vi "grabAcquire_action.vi"(0 "HGF_ImaqDx":refnum<class "HGF_ImaqDx.lvclass">, 2 "Image In":T1, 3 "Wait for Next Buffer? (Yes)":bool=TRUE, 5 "error in (no error)":errorcluster) -> (14 "dup HGF_ImaqDx":refnum<class "HGF_ImaqDx.lvclass">, 16 "Image Out":T1, 17 "Acquired Buffer Number":u32, 19 "error out":errorcluster)   [LabVIEW 2014, in "HGF_IMAQ.lvlib" / "HGF_ImaqDx.lvclass"]
doc: "Acquires an image from a grab acquisition. Use the grab function for high-speed image acquisition.\n\nWait parameter is ignored by IMAQ for USB."
uses:
  HGF_ImaqDx.lvclass
  <vilib>/vision/Image Controls.llb/IMAQ Image.ctl
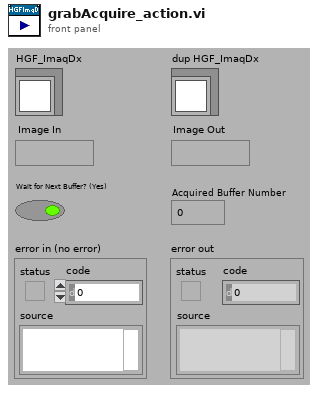
[diagram p1: front panel]
types:
  T1 = typedef "IMAQ Image.ctl" = refnum<image>
  T2 = typedef "IMAQdx.ctl" = refnum<k21>
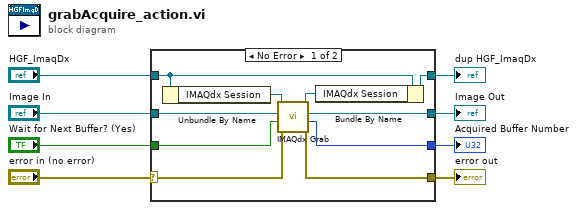
[diagram p0: block diagram]
diagram:
  n1 = case shown="No Error" "error in (no error)" {
    selector: "error in (no error)" -> [w9 w19]
    tunnel: "Image In" -> [w18 w20]
    tunnel: [w17 w20] -> w7
    tunnel: "Wait for Next Buffer? (Yes)" -> [w16 _]
    tunnel: [w15 _] -> w5
    tunnel: "HGF_ImaqDx" -> [w13 w21]
    tunnel: [w12 w21] -> w3
    tunnel: [w10 w19] -> w2
    frame No Error {
      n2 = Unbundle By Name(w13) -> ("IMAQdx Session"=w14:T2)
      n3 = call <vilib>:"IMAQdx Grab.vi"("error in"=w9, "Wait for Next Buffer? (Yes)"=w16, "Image In"=w18, "Session In"=w14) -> ("error out"=w10:errorcluster, "Buffer Number Out"=w15:u32, "Image Out"=w17:T1, "Session Out"=w11:T2)  [unwired: 4 out]
      n4 = Bundle By Name(cluster=w13, "IMAQdx Session"=w11) -> (w12:refnum<class "HGF_ImaqDx.lvclass">)
    }
    frame Error {
    }
  }
  "error out" <- w2
  "dup HGF_ImaqDx" <- w3
  "Image Out" <- w7
  "Acquired Buffer Number" <- w5
